vi "UEGO Calibration States to Word.vi"(11 "UEGO Calibration States":T1) -> (3 "UEGO Calibration Word":u16 format="%016b")   [LabVIEW 2014, in "SLSC configuration Shared.lvlib"]
doc: "Converts four faults to a fault word."
uses:
  SLSC configuration Shared.lvlib
  Bank Calibration States.ctl
  Calibration State.ctl
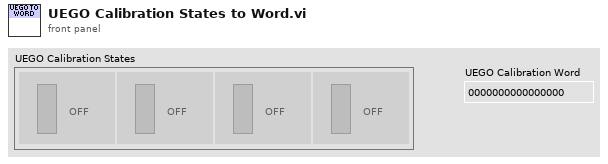
[diagram p1: front panel]
types:
  T1 = typedef "SLSC configuration Shared.lvlib/Bank Calibration States.ctl" = T2[]
  T2 = typedef "SLSC configuration Shared.lvlib/Calibration State.ctl" = bool
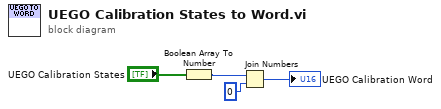
[diagram p0: block diagram]
diagram:
  n1 = Boolean Array To Number(Boolean array="UEGO Calibration States") -> (number=w2:u8)
  n2 = Join Numbers(hi=w2, lo=u8 0) -> ((hi.lo)=→"UEGO Calibration Word":u16)
